vi "Configure Receiver Calibration.vi"(7 "Channel (1)":i32=1, 8 "error in (no error)":errorcluster, 9 "Receiver Correction State (F: Disabled)":bool, 10 "Receiver (1)":i32=1, 11 "VISA resource name":refnum<visa-resource-name>) -> (0 "error out":errorcluster, 3 "VISA resource name out":refnum<visa-resource-name>)   [LabVIEW 2020, in "Agilent ENA Series.lvlib"]
doc: "Enables or disables the receiver correction.\n\n<b>Note:</b>\nThis VI is not supported by the E5063A, E5080A and E5080B model."
uses:
  <instrlib>/Agilent ENA Series/Agilent ENA Series.lvlib
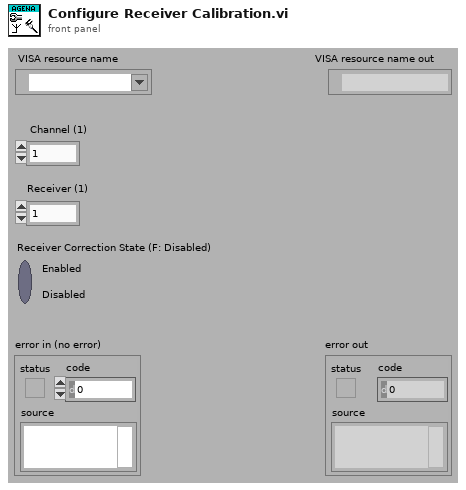
[diagram p1: front panel]
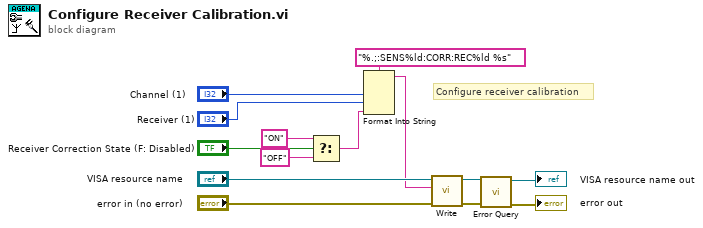
[diagram p0: block diagram]
diagram:
  # "Configure receiver calibration"
  n1 = Select(t="ON", s="Receiver Correction State (F: Disabled)", f="OFF") -> (s? t:f=w6:string)
  n2 = Format Into String(format string="%.;:SENS%ld:CORR:REC%ld %s", "Channel (1)", "Receiver (1)", w6) -> (resulting string=w5:string)  [unwired: 2 in, 1 out]
  n3 = call <instrlib>:"Write.vi"("error in (no error)"="error in (no error)", "String ()"=w5, "VISA resource name"="VISA resource name") -> ("error out"=w3:errorcluster, "VISA resource name out"=w4:refnum<visa-resource-name>)  [unwired: 6 in, 1 out]
  n4 = call <instrlib>:"Error Query.vi"("error in (no error)"=w3, "VISA resource name"=w4) -> ("error out"=→"error out":errorcluster, "VISA resource name out"=→"VISA resource name out":refnum<visa-resource-name>)  [unwired: 6 in, 2 out]
